vi "Get GCD.vi"(7 "Within":dbl=0.1 format="%#_13g", 10 "Y":dbl, 11 "X":dbl) -> (3 "GCD":dbl)   [LabVIEW 2019, in "Tool Rectangle.lvclass"]
uses:
  Tool Rectangle.lvclass
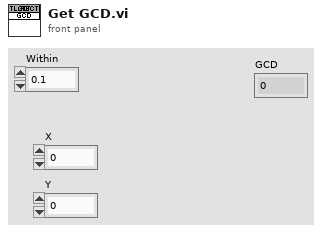
[diagram p1: front panel]
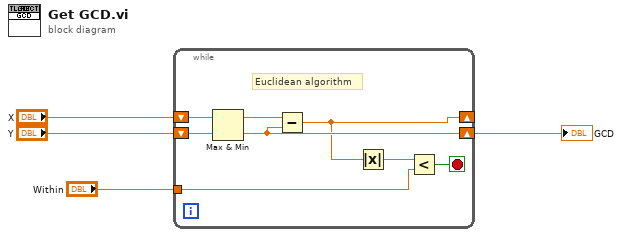
[diagram p0: block diagram]
diagram:
  n1 = while {
    shift-right: [w5] -> _
    shift-left: "X" -> [w10]
    shift-right: [w6] -> w1
    shift-left: "Y" -> [w12]
    tunnel: "Within" -> [w8]
    stop <- w9 stop-if-true
    # "Euclidean algorithm"
    n2 = Max & Min(x=w10, y=w12) -> (max(x,y)=w11:dbl, min(x,y)=w6:dbl)
    n3 = Subtract(x=w11, y=w6) -> (x-y=w5:dbl)
    n4 = Absolute Value(x=w5) -> (abs(x)=w7:dbl)
    n5 = Less?(x=w7, y=w8) -> (x < y?=w9:bool)
  }
  "GCD" <- w1
